vi "op_biti_v7.vi"() -> ()   [LabVIEW 2009]
panel:
  out "C=A AND B":dbl=85.0
  out "B":dbl=255.0
  out "A":dbl=85.0
  out "Array 5":bool[](array[boolean])=[FALSE, TRUE, FALSE, TRUE, FALSE, TRUE, FALSE, TRUE]
  in  "Array 4":bool[](array[boolean])=[TRUE, TRUE, TRUE, TRUE, TRUE, TRUE, TRUE, TRUE]
  out "Array 3":bool[](array[boolean])=[TRUE, TRUE, TRUE, TRUE, TRUE, TRUE, TRUE, TRUE]
  in  "Array 2":bool[](array[boolean])=[FALSE, TRUE, FALSE, TRUE, FALSE, TRUE, FALSE, TRUE]
  out "Array":bool[](array[boolean])=[FALSE, TRUE, FALSE, TRUE, FALSE, TRUE, FALSE, TRUE]
  # "A"
  # "B"
  # "C=A AND B"
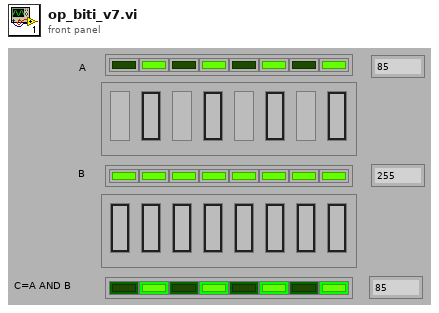
[diagram p1: front panel]
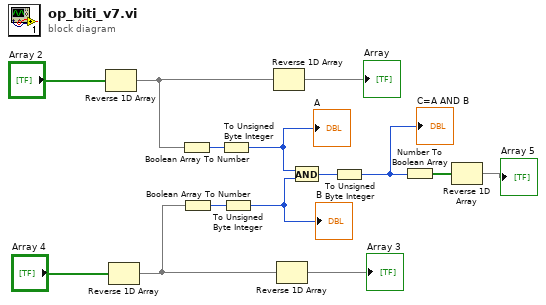
[diagram p0: block diagram]
diagram:
  n1 = Reverse 1D Array(array="Array 2") -> (reversed array=w13:bool[])
  n2 = Reverse 1D Array(array="Array 4") -> (reversed array=w10:bool[])
  n3 = Boolean Array To Number(Boolean array=w13) -> (number=w6:u32)
  n4 = Boolean Array To Number(Boolean array=w10) -> (number=w5:u32)
  n5 = To Unsigned Byte Integer(number=w6) -> (unsigned 8bit integer=w4:u8)
  "A" <- w4
  n6 = To Unsigned Byte Integer(number=w5) -> (unsigned 8bit integer=w3:u8)
  "B" <- w3
  n7 = Reverse 1D Array(array=w13) -> (reversed array=→"Array":bool[])
  n8 = Reverse 1D Array(array=w10) -> (reversed array=→"Array 3":bool[])
  n9 = And(x=w4, y=w3) -> (x .and. y?=w2:u8)
  n10 = To Unsigned Byte Integer(number=w2) -> (unsigned 8bit integer=w1:u8)
  "C=A AND B" <- w1
  n11 = Number To Boolean Array(number=w1) -> (Boolean array=w8:bool[])
  n12 = Reverse 1D Array(array=w8) -> (reversed array=→"Array 5":bool[])
